vi "Throw Unsupported Sweep Settings Error.vi"(0 "Error Message List":string[](array[string]), 5 "Delimiter ('\\n')":string="\n", 7 "Additional Header":string, 9 "Additional Details":string, 11 "error in":errorcluster) -> (15 "error out":errorcluster)   [LabVIEW 2023, in "RFCalAndFixtureCharact.Common.lvlib"]
uses:
  RFCalAndFixtureCharact.Common.lvlib
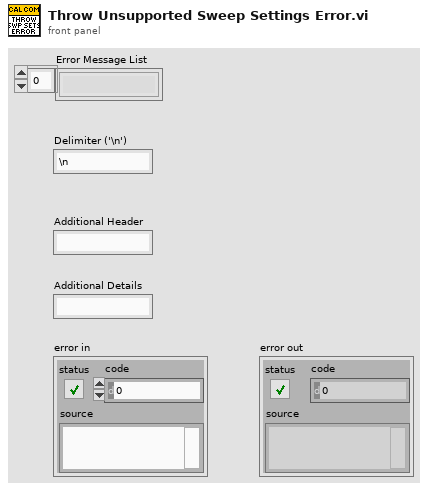
[diagram p1: front panel]
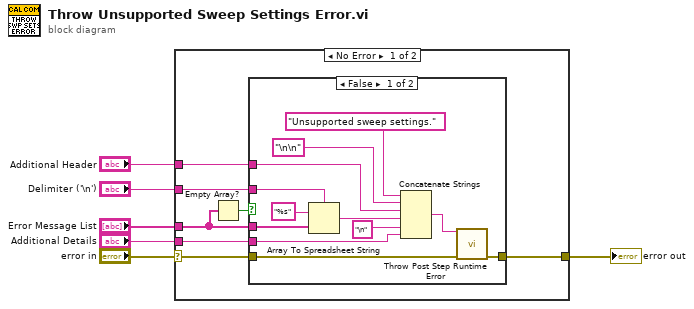
[diagram p0: block diagram]
diagram:
  n1 = case shown="No Error" "error in" {
    selector: "error in" -> [w12 w27]
    tunnel: "Error Message List" -> [w10 _]
    tunnel: [w13 w27] -> w5
    tunnel: "Delimiter ('\\n')" -> [w9 _]
    tunnel: "Additional Header" -> [w8 _]
    tunnel: "Additional Details" -> [w7 _]
    frame No Error {
      n2 = Empty Array?(array=w10) -> (empty?=w11:bool)
      n3 = case shown="False" w11 {
        tunnel: w10 -> [w24 _]
        tunnel: [w23 w26] -> w13
        tunnel: w12 -> [w20 w26]
        tunnel: w9 -> [w19 _]
        tunnel: w8 -> [w16 _]
        tunnel: w7 -> [w17 _]
        frame False {
          n4 = Array To Spreadsheet String(delimiter (Tab)=w19, array=w24, 3:"%s" ("format string")) -> (spreadsheet string=w22:string)
          n5 = Concatenate Strings("Unsupported sweep settings.", "\n\n" ("string"), w16, w22, "\n" ("string"), w17) -> (w21:string)
          n6 = call "Throw Post Step Runtime Error.vi"("Error Message"=w21, "error in"=w20) -> ("error out"=w23:errorcluster)  [unwired: 13 in]
        }
        frame True {
        }
      }
    }
    frame Error {
    }
  }
  "error out" <- w5
